vi "Initialize.vi"(8 "error in (no error)":errorcluster, 9 "Serial Settings Additional":T1={"termination char\n(0xA = '\\n' = LF) "=10, "Enable Termination\nChar (T)"=FALSE, "timeout (10sec)"=10000} {"termination char\n(0xA = '\\n' = LF)" format="%.0x"}, 10 "Serial Settings":T2={"baud rate"=115200, "data bits"=8, "parity"=enum."None", "stop bits"=10, "flow control"=0} {"flow control" items=["None"=0, "XON/XOFF"=1, "RTS/CTS"=2, "DTR/DSR"=4]; "stop bits" items=["1.0"=10, "1.5"=15, "2.0"=20]; "data bits" min=5 max=8 step=1; "baud rate" items=["75"=75, "110"=110, "134"=134, "150"=150, "300"=300, "600"=600, "1200"=1200, "1800"=1800, "2400"=2400, "4800"=4800, "7200"=7200, "9600"=9600, "14400"=14400, "19200"=19200, "28800"=28800, "38400"=38400, "56000"=56000, "57600"=57600, "115200"=115200, "128000"=128000, "230400"=230400]}, 11 "VISA resource name":refnum<visa-resource-name>) -> (0 "error out":errorcluster, 3 "VISA resource name":refnum<visa-resource-name>)   [LabVIEW 2025]
uses:
  <vilib>/Instr/_visa.llb/VISA Configure Serial Port (Instr).vi
  <vilib>/Serial Port/Type Definitions/Serial Settings.ctl
  <vilib>/Serial Port/SerialPort.lvlib
  <vilib>/Serial Port/Type Definitions/Serial Settings Additional.ctl
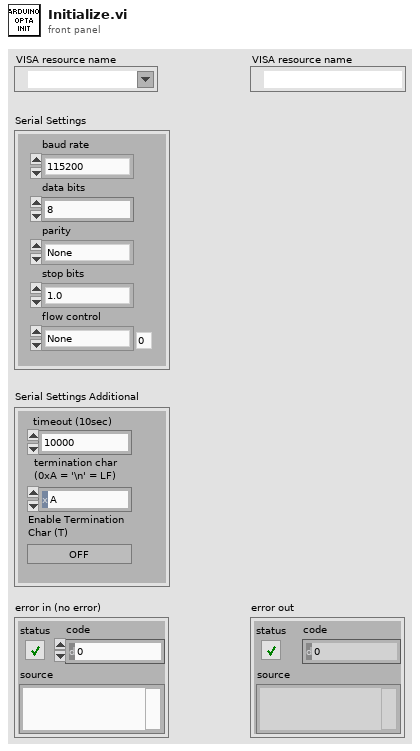
[diagram p1: front panel]
types:
  T1 = typedef "SerialPort.lvlib/Serial Settings Additional.ctl" = cluster{"termination char\n(0xA = '\\n' = LF) ":u8, "Enable Termination\nChar (T)":bool, "timeout (10sec)":u32}
  T2 = typedef "SerialPort.lvlib/Serial Settings.ctl" = cluster{"baud rate":u32, "data bits":u16, "parity":enum16{"None", "Odd", "Even", "Mark", "Space"}, "stop bits":u16, "flow control":u16}
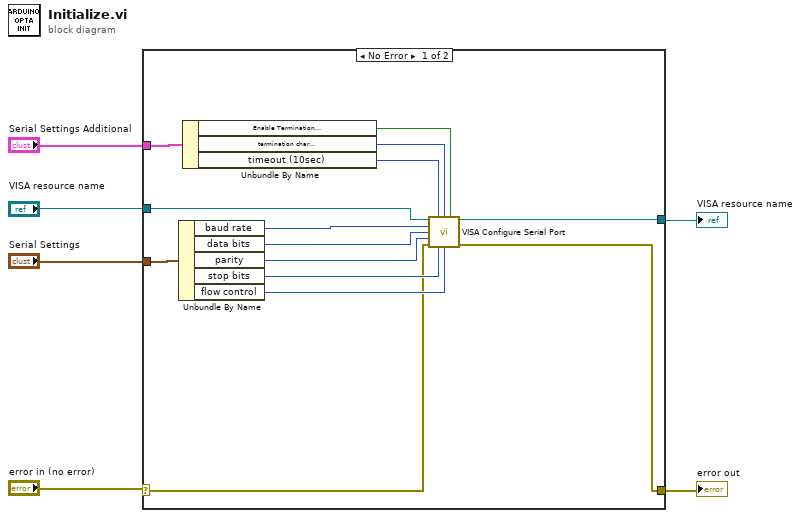
[diagram p0: block diagram]
diagram:
  n1 = case shown="No Error" "error in (no error)" {
    selector: "error in (no error)" -> [w11 w22]
    tunnel: "Serial Settings" -> [w20 _]
    tunnel: "VISA resource name" -> [w14 w21]
    tunnel: "Serial Settings Additional" -> [w13 _]
    tunnel: [w12 w22] -> w2
    tunnel: [w7 w21] -> w1
    frame No Error {
      n2 = Unbundle By Name(w20) -> ("baud rate"=w19:u32, "data bits"=w18:u16, "parity"=w17:enum16{"None", "Odd", "Even", "Mark", "Space"}, "stop bits"=w16:u16, "flow control"=w15:u16)
      n3 = Unbundle By Name(w13) -> ("Enable Termination\nChar (T)"=w9:bool, "termination char\n(0xA = '\\n' = LF)"=w8:u8, "timeout (10sec)"=w10:u32)
      n4 = call-poly "VISA Configure Serial Port"("VISA resource name"=w14, "timeout (10sec)"=w10, "termination char\n(0xA = '\\n' = LF)"=w8, "Enable Termination\nChar (T)"=w9, "baud rate (9600)"=w19, "data bits (8)"=w18, "parity (0:none)"=w17, "error in (no error)"=w11, "stop bits (10: 1 bit)"=w16, "flow control (0:none)"=w15) -> ("VISA resource name out"=w7:refnum<visa-resource-name>, "error out"=w12:errorcluster)  [unwired: 4 out]
    }
    frame Error {
    }
  }
  "error out" <- w2
  "VISA resource name" <- w1
